vi "serialization test.vi"() -> ()   [LabVIEW 2013, in "std eng tests.lvlib"]
uses:
  std eng tests.lvlib
  Runtime/Standard Engine Runtime.lvclass
  <vilib>/NI/Tag Bus Module Framework/channel/channel classification.ctl
  <vilib>/NI/Tag Bus/tag/Data Type.ctl
  Configuration/Module Decimation.ctl
  Configuration/Supported Timing Sources.ctl
  testmodule/execution/testmod runtime.lvclass
  testmodule/configuration/testmod configuration.lvclass
  Configuration/timing reporting tags.ctl
  Configuration/Standard Engine Configuration.lvclass
  Runtime/error responses.ctl
  Configuration/error options.ctl
  Configuration/Standard Engine Configuration.lvclass/Standard Engine Configuration.ctl
  <vilib>/NI/Tag Bus/tag/tag descriptor.lvclass
  Configuration/Write Timing Source Type.vi
  Configuration/Read Master Timing Module.vi
  Configuration/Read Processor.vi
  Configuration/Read timing policy.vi
  Configuration/Read Timing Source Type.vi
  Configuration/Write Timing Source dt.vi
  Configuration/Find Module Specific Config.vi
  <vilib>/NI/Configuration Framework/error generator.vi
  Configuration/Read Timing Source dt.vi
  <vilib>/NI/Tag Bus Module Framework/channel/TBM channel.lvclass
  <vilib>/NI/Module Execution Interface/Engine Configuration/engine configuration.lvclass
  <vilib>/NI/Configuration Framework/serializable configuration/NISE_CEF_serializable configuration.lvclass
panel:
  out "Array":T1(array[cluster])
  out "x = y?":T2(array[cluster])
  out "serialization ok 7":bool
  out "serialization ok 6":bool
  out "serialization ok 5":bool
  out "serialization ok 4":bool
  out "serialization ok 3":bool
  out "ALL OK":bool
  out "errrrr":errorcluster
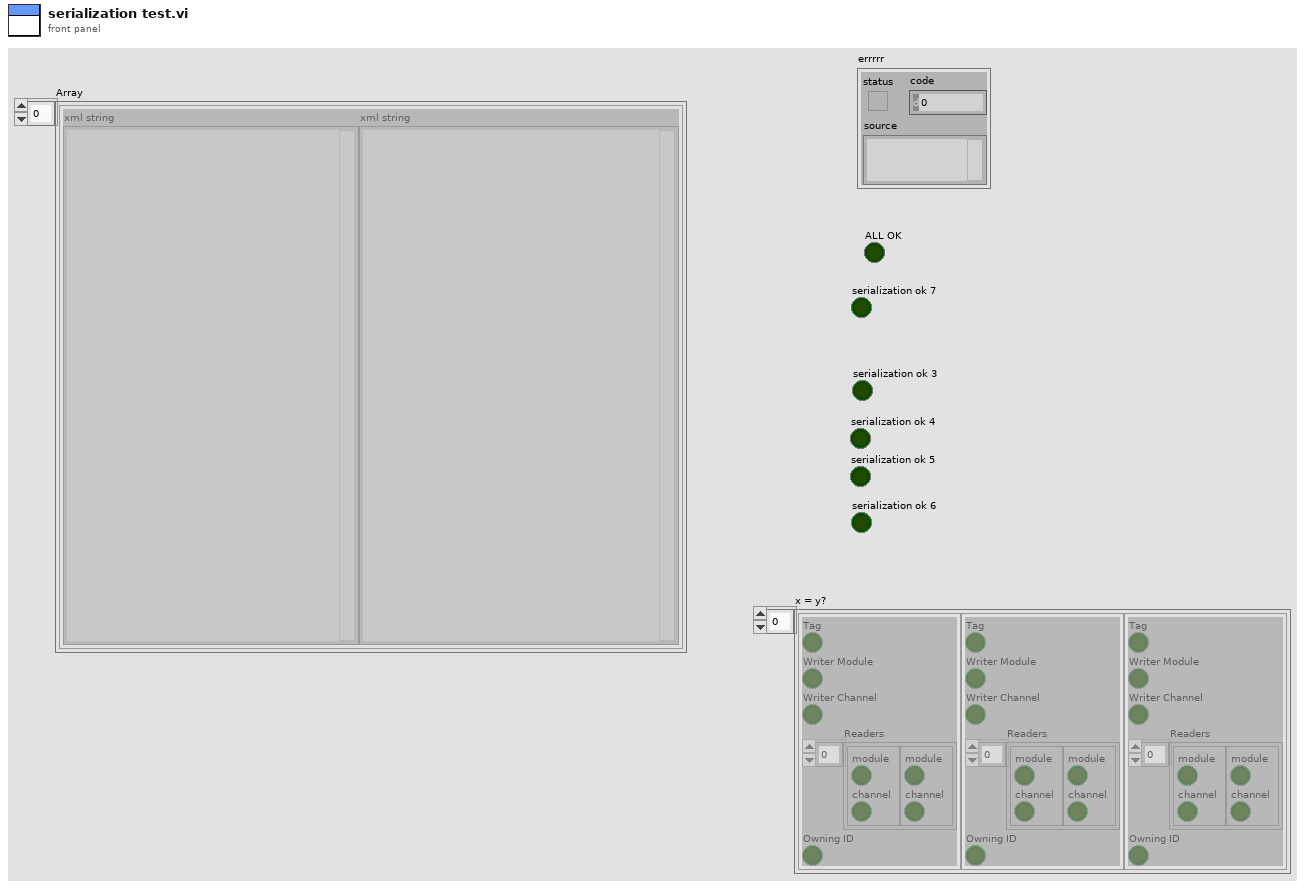
[diagram p1: front panel]
types:
  T1 = cluster{"xml string":string, "xml string":string}[]
  T2 = cluster{"Tag":bool, "Writer Module":bool, "Writer Channel":bool, "Readers":cluster{"module":bool, "channel":bool}[], "Owning ID":bool}[]
  T3 = typedef "Standard Engine Configuration.lvclass/error responses.ctl" = cluster{"unknown":T4, "trivial":T4, "critical":T4, "recoverable":T4}
  T4 = typedef "Standard Engine Configuration.lvclass/error options.ctl" = cluster{"clear":bool, "notify":bool, "remove module":bool, "abort engine":bool, "go to safe state":bool, "recover module":bool}
  T5 = typedef "Standard Engine Configuration.lvclass/timing reporting tags.ctl" = cluster{"late index (bool)":string, "late count index (U32)":string, "current dt ns(U64)":string}
  T6 = typedef "tag bus.lvlib/tag descriptor.lvclass/Data Type.ctl" = enum16{"Double", "Single", "I64", "I32", "I16", "I8", "U64", "U32", "U16", "U8", "Boolean", "String", "Array of Double", "Array of Single", "Array of I64", "Array of I32", "Array of I16", "Array of I8", "Array of U64", "Array of U32", "Array of U16", "Array of U8", "Array of Boolean", "Array of String"}
  T7 = typedef "TBM channel.lvclass/channel classification.ctl" = enum16{"input data", "output data", "processing parameter", "processing result"}
  T8 = typedef "Standard Engine Configuration.lvclass/Supported Timing Sources.ctl" = enum16{"Use Module Timing Source", "1 kHz Clock", "1 MHz Clock", "Synchronize to Scan Engine"}
  T9 = typedef "Standard Engine Configuration.lvclass/Module Decimation.ctl" = cluster{"Decimation":u16, "Offset":u16, "sort order":i32, "async?":bool}
  T10 = typedef "engine configuration.lvclass/Tag Info.ctl" = cluster{"Tag":refnum<class "tag descriptor.lvclass">, "Writer Module":string, "Writer Channel":string, "Readers":cluster{"module":string, "channel":string}[], "Owning ID":string}
  T11 = typedef "Standard Engine Configuration.lvclass/timing policy.ctl" = enum16{"strict determinism", "nonblocking", "nondeterministic inline"}
  T12 = cluster{"xml string":string, "xml string":string}
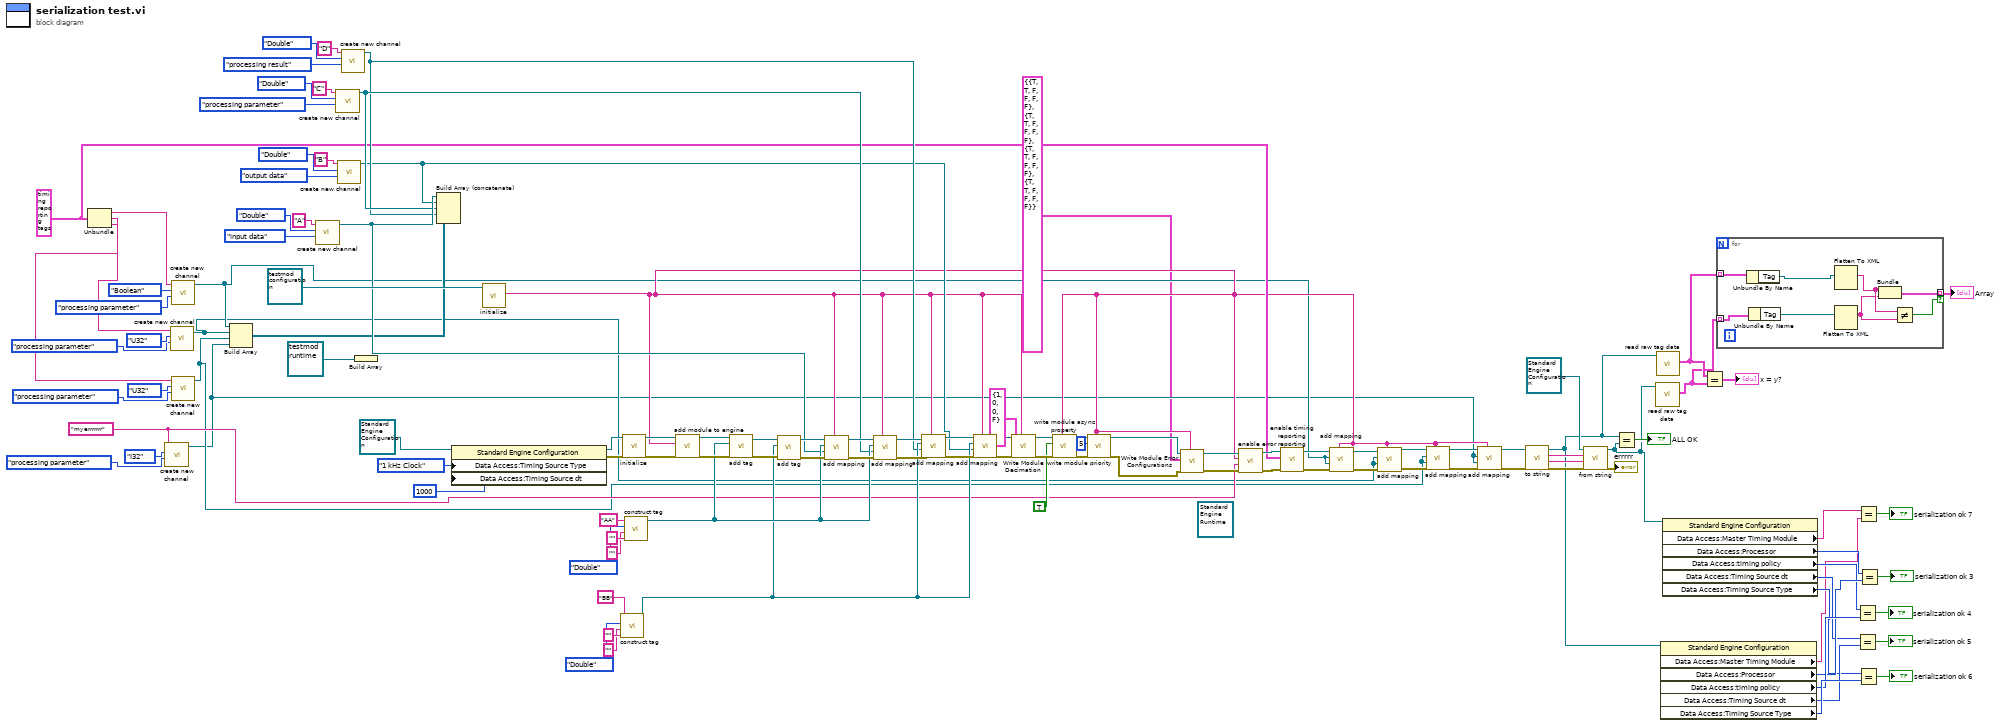
[diagram p0: block diagram]
diagram:
  w44 = T5 {"late index (bool)"="late", "late count index (U32)"="lcount", "current dt ns(U64)"="dt"} ("timing reporting")
  w45 = "myerrrrrrr" ("channel name")
  (unwired) refnum<class "Standard Engine Runtime.lvclass"> refnum ("Standard Engine Runtime")
  n1 = Unbundle(w44) -> ("late index (bool)"=w51:string, "late count index (U32)"=w50:string, "current dt ns(U64)"=w49:string)
  n2 = call <vilib>:"create new channel.vi"("channel classification"=channel_classification."processing parameter", "data type"=Data_Type."I32", "channel name"=w45) -> ("channel"=w31:refnum<class "TBM channel.lvclass">)  [unwired: 8 in]
  n3 = call <vilib>:"create new channel.vi"("channel classification"=channel_classification."processing parameter", "data type"=Data_Type."U32", "channel name"=w50) -> ("channel"=w33:refnum<class "TBM channel.lvclass">)  [unwired: 8 in]
  n4 = call <vilib>:"create new channel.vi"("channel classification"=channel_classification."processing parameter", "data type"=Data_Type."Boolean", "channel name"=w51) -> ("channel"=w34:refnum<class "TBM channel.lvclass">)  [unwired: 8 in]
  n5 = call <vilib>:"create new channel.vi"("channel classification"=channel_classification."processing parameter", "data type"=Data_Type."U32", "channel name"=w49) -> ("channel"=w32:refnum<class "TBM channel.lvclass">)  [unwired: 8 in]
  n6 = Build Array(w34, w33, w32, w31) -> (w46:refnum<class "TBM channel.lvclass">[])
  n7 = call <vilib>:"create new channel.vi"("channel classification"=channel_classification."input data", "data type"=Data_Type."Double", "channel name"="A") -> ("channel"=w67:refnum<class "TBM channel.lvclass">)  [unwired: 8 in]
  n8 = call <vilib>:"create new channel.vi"("channel classification"=channel_classification."processing parameter", "data type"=Data_Type."Double", "channel name"="C") -> ("channel"=w66:refnum<class "TBM channel.lvclass">)  [unwired: 8 in]
  n9 = call <vilib>:"create new channel.vi"("channel classification"=channel_classification."output data", "data type"=Data_Type."Double", "channel name"="B") -> ("channel"=w64:refnum<class "TBM channel.lvclass">)  [unwired: 8 in]
  n10 = call <vilib>:"create new channel.vi"("channel classification"=channel_classification."processing result", "data type"=Data_Type."Double", "channel name"="D") -> ("channel"=w65:refnum<class "TBM channel.lvclass">)  [unwired: 8 in]
  n11 = Build Array(refnum<class "testmod runtime.lvclass"> refnum ("CVT runtime")) -> ()  [unwired: 1 out]
  n12 = Build Array (concatenate)(w67, w64, w66, w65, w46) -> ()  [unwired: 1 out]
  n13 = property class="Standard Engine Configuration"(reference=refnum<class "Standard Engine Configuration.lvclass"> refnum ("Standard Engine Configuration"), "Data Access:Timing Source Type"=Supported_Timing_Sources."1 kHz Clock" ("Timing Source Type"), "Data Access:Timing Source dt"=u32 1000 ("Timing Source dt")) -> (reference out=w96:refnum<class "Standard Engine Configuration.lvclass">, error out=w98:errorcluster)  [unwired: 1 in]
  n14 = call <vilib>:"initialize.vi"("configuration in"=refnum<class "testmod configuration.lvclass"> refnum ("CVT configuration")) -> ("identifier"=w35:string)  [unwired: 8 in, 2 out]
  n15 = call <vilib>:"construct tag.vi"("raw default"="", "metadata"="", "data type"=Data_Type."Double", "name"="BB") -> ("system tag out"=w68:refnum<class "tag descriptor.lvclass">)  [unwired: 6 in, 1 out]
  n16 = call <vilib>:"initialize.vi"("error in"=w98, "configuration in"=w96) -> ("error out"=w109:errorcluster, "configuration out"=w108:refnum<class "Standard Engine Configuration.lvclass">)  [unwired: 7 in, 1 out]
  n17 = call <vilib>:"construct tag.vi"("raw default"="", "metadata"="", "data type"=Data_Type."Double", "name"="AA") -> ("system tag out"=w69:refnum<class "tag descriptor.lvclass">)  [unwired: 6 in, 1 out]
  n18 = call-dynamic "add module to engine.vi"("error in"=w109, "module ID"=w35, "Standard Engine Configuration in"=w108) -> ("error out"=w111:errorcluster, "Standard Engine Configuration out"=w110:refnum<class "Standard Engine Configuration.lvclass">)  [unwired: 7 in]
  n19 = call <vilib>:"add tag.vi"("error in"=w111, "tag descriptor"=w69, "engine configuration in"=w110) -> ("error out"=w84:errorcluster, "engine configuration out"=w85:refnum<class "Standard Engine Configuration.lvclass">)  [unwired: 7 in]
  n20 = call <vilib>:"add tag.vi"("error in"=w84, "tag descriptor"=w68, "engine configuration in"=w85) -> ("error out"=w83:errorcluster, "engine configuration out"=w71:refnum<class "Standard Engine Configuration.lvclass">)  [unwired: 7 in]
  n21 = call <vilib>:"add mapping.vi"("owner ID"=w35, "error in"=w83, "channel"=w67, "tag descriptor"=w69, "engine configuration"=w71) -> ("error out"=w72:errorcluster, "engine configuration out"=w70:refnum<class "Standard Engine Configuration.lvclass">)  [unwired: 5 in]
  n22 = call <vilib>:"add mapping.vi"("owner ID"=w35, "error in"=w72, "channel"=w66, "tag descriptor"=w69, "engine configuration"=w70) -> ("error out"=w74:errorcluster, "engine configuration out"=w73:refnum<class "Standard Engine Configuration.lvclass">)  [unwired: 5 in]
  n23 = call <vilib>:"add mapping.vi"("owner ID"=w35, "error in"=w74, "channel"=w65, "tag descriptor"=w68, "engine configuration"=w73) -> ("error out"=w113:errorcluster, "engine configuration out"=w112:refnum<class "Standard Engine Configuration.lvclass">)  [unwired: 5 in]
  n24 = call <vilib>:"add mapping.vi"("owner ID"=w35, "error in"=w113, "channel"=w64, "tag descriptor"=w68, "engine configuration"=w112) -> ("error out"=w104:errorcluster, "engine configuration out"=w105:refnum<class "Standard Engine Configuration.lvclass">)  [unwired: 5 in]
  n25 = call "Write Module Decimation.vi"("Module ID"=w35, "error in"=w104, "Module Decimation"=T9 {"Decimation"=1, "Offset"=0, "sort order"=0, "async?"=FALSE}, "Standard Engine Repo Data in"=w105) -> ("error out"=w106:errorcluster, "Standard Engine Repo Data out"=w107:refnum<class "Standard Engine Configuration.lvclass">)  [unwired: 6 in]
  n26 = call "write module async property.vi"("Module ID"=w35, "error in"=w106, "async?"=TRUE, "Standard Engine Repo Data in"=w107) -> ("error out"=w103:errorcluster, "Standard Engine Repo Data out"=w102:refnum<class "Standard Engine Configuration.lvclass">)  [unwired: 6 in]
  n27 = call "write module priority.vi"("Module ID"=w35, "error in"=w103, "execution order priority"=5, "Standard Engine Repo Data in"=w102) -> ("error out"=w58:errorcluster, "Standard Engine Repo Data out"=w63:refnum<class "Standard Engine Configuration.lvclass">)  [unwired: 6 in]
  n28 = call "Write Module Error Configurations.vi"("Module ID"=w35, "error in"=w58, "error responses"=T3 {"unknown"={"clear"=TRUE, "notify"=TRUE, "remove module"=FALSE, "abort engine"=FALSE, "go to safe state"=FALSE, "recover module"=FALSE}, "trivial"={"clear"=TRUE, "notify"=TRUE, "remove module"=FALSE, "abort engine"=FALSE, "go to safe state"=FALSE, "recover module"=FALSE}, "critical"={"clear"=TRUE, "notify"=TRUE, "remove module"=FALSE, "abort engine"=FALSE, "go to safe state"=FALSE, "recover module"=FALSE}, "recoverable"={"clear"=TRUE, "notify"=TRUE, "remove module"=FALSE, "abort engine"=FALSE, "go to safe state"=FALSE, "recover module"=FALSE}}, "Standard Engine Repo Data in"=w63) -> ("error out"=w59:errorcluster, "Standard Engine Repo Data out"=w62:refnum<class "Standard Engine Configuration.lvclass">)  [unwired: 6 in]
  n29 = call "enable error reporting.vi"("error in"=w59, "tag"=w45, "module ID"=w35, "Standard Engine Configuration in"=w62) -> ("error out"=w60:errorcluster, "Standard Engine Configuration out"=w61:refnum<class "Standard Engine Configuration.lvclass">)  [unwired: 6 in]
  n30 = call "enable timing reporting.vi"("error in"=w60, "timing reporting"=w44, "Standard Engine Configuration in"=w61) -> ("error out"=w36:errorcluster, "Standard Engine Configuration out"=w37:refnum<class "Standard Engine Configuration.lvclass">)  [unwired: 7 in]
  n31 = call <vilib>:"add mapping.vi"("owner ID"=w35, "error in"=w36, "channel"=w34, "tag descriptor"=w34, "engine configuration"=w37) -> ("error out"=w42:errorcluster, "engine configuration out"=w43:refnum<class "Standard Engine Configuration.lvclass">)  [unwired: 5 in]
  n32 = call <vilib>:"add mapping.vi"("owner ID"=w35, "error in"=w42, "channel"=w33, "tag descriptor"=w33, "engine configuration"=w43) -> ("error out"=w40:errorcluster, "engine configuration out"=w41:refnum<class "Standard Engine Configuration.lvclass">)  [unwired: 5 in]
  n33 = call <vilib>:"add mapping.vi"("owner ID"=w35, "error in"=w40, "channel"=w32, "tag descriptor"=w32, "engine configuration"=w41) -> ("error out"=w38:errorcluster, "engine configuration out"=w39:refnum<class "Standard Engine Configuration.lvclass">)  [unwired: 5 in]
  n34 = call <vilib>:"add mapping.vi"("owner ID"=w35, "error in"=w38, "channel"=w31, "tag descriptor"=w31, "engine configuration"=w39) -> ("error out"=w29:errorcluster, "engine configuration out"=w28:refnum<class "Standard Engine Configuration.lvclass">)  [unwired: 5 in]
  n35 = call-dynamic "to string.vi"("error in"=w29, "Standard Engine Repo Data in"=w28) -> ("error out"=w30:errorcluster, "data"=w26:string, "version"=w27:string, "Standard Engine Repo Data out"=w6:refnum<class "Standard Engine Configuration.lvclass">)  [unwired: 6 in]
  n36 = call-dynamic "from string.vi"("error in"=w30, "data"=w26, "version"=w27, "Standard Engine Repo Data in"=refnum<class "Standard Engine Configuration.lvclass"> refnum ("Standard Engine Configuration")) -> ("error out"=→"errrrr":errorcluster, "Standard Engine Repo Data out"=w7:refnum<class "Standard Engine Configuration.lvclass">)  [unwired: 6 in]
  n37 = Equal?(x=w6, y=w7) -> (x = y?=→"ALL OK":bool)
  n38 = call <vilib>:"read raw tag data.vi"("engine configuration in"=w7) -> ("raw tag data"=w3:T10[])  [unwired: 8 in, 2 out]
  n39 = call <vilib>:"read raw tag data.vi"("engine configuration in"=w6) -> ("raw tag data"=w4:T10[])  [unwired: 8 in, 2 out]
  n40 = property class="Standard Engine Configuration"(reference=w6) -> ("Data Access:Master Timing Module"=w8:string, "Data Access:Processor"=w15:i32, "Data Access:timing policy"=w16:T11, "Data Access:Timing Source dt"=w17:u32, "Data Access:Timing Source Type"=w18:T8)  [unwired: 1 in, 2 out]
  n41 = property class="Standard Engine Configuration"(reference=w7) -> ("Data Access:Master Timing Module"=w9:string, "Data Access:Processor"=w14:i32, "Data Access:timing policy"=w13:T11, "Data Access:Timing Source dt"=w12:u32, "Data Access:Timing Source Type"=w11:T8)  [unwired: 1 in, 2 out]
  n42 = Equal?(x=w4, y=w3) -> (x = y?=→"x = y?":T2)
  n43 = for {
    tunnel: w4 -> [w127] mode=indexing
    tunnel: w3 -> [w126] mode=indexing
    tunnel: [w123] -> w2 mode=indexing if=w120
    n44 = Unbundle By Name(w127) -> ("Tag"=w125:refnum<class "tag descriptor.lvclass">)
    n45 = Unbundle By Name(w126) -> ("Tag"=w124:refnum<class "tag descriptor.lvclass">)
    n46 = Flatten To XML(anything=w125) -> (xml string=w122:string)
    n47 = Flatten To XML(anything=w124) -> (xml string=w121:string)
    n48 = Bundle("xml string"=w122, "xml string"=w121) -> (w123:T12)  [unwired: 1 in]
    n49 = Not Equal?(x=w122, y=w121) -> (x != y?=w120:bool)
  }
  "Array" <- w2
  n50 = Equal?(x=w13, y=w16) -> (x = y?=→"serialization ok 4":bool)
  n51 = Equal?(x=w12, y=w17) -> (x = y?=→"serialization ok 5":bool)
  n52 = Equal?(x=w9, y=w8) -> (x = y?=→"serialization ok 7":bool)
  n53 = Equal?(x=w11, y=w18) -> (x = y?=→"serialization ok 6":bool)
  n54 = Equal?(x=w14, y=w15) -> (x = y?=→"serialization ok 3":bool)
